vi "8_ВПАнализСтрок.vi"() -> ()   [LabVIEW 2016]
panel:
  out "No Match":bool
  out "Matched Pattern":string
  in  "Password":string
  out "String Subset":string
  in  "Input String":string
  out "Number":dbl
  in  "Number Offset":i16
  in  "Subset Length":i16
  in  "Subset Offset":i16
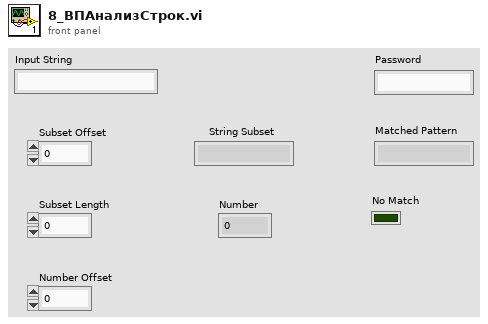
[diagram p1: front panel]
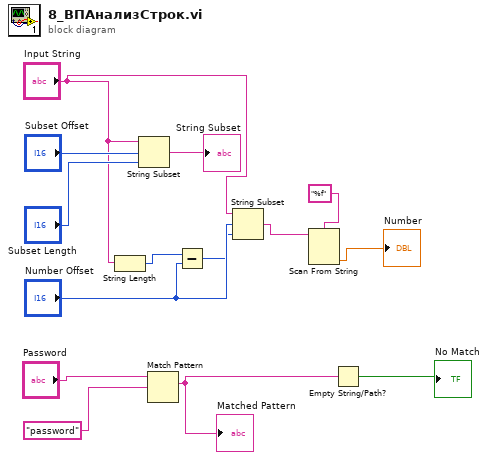
[diagram p0: block diagram]
diagram:
  n1 = String Length(string="Input String") -> (length=w3:i32)
  n2 = String Subset(string="Input String", offset (0)="Subset Offset", length (rest)="Subset Length") -> (substring=→"String Subset":string)
  n3 = Match Pattern(string="Password", regular expression="password") -> (match substring=w5:string)  [unwired: 1 in, 3 out]
  "Matched Pattern" <- w5
  n4 = Subtract(x=w3, y="Number Offset") -> (x-y=w1:i32)
  n5 = String Subset(string="Input String", offset (0)="Number Offset", length (rest)=w1) -> (substring=w10:string)
  n6 = Scan From String(format string="%f", input string=w10) -> (output 1=→"Number":dbl)  [unwired: 3 in, 3 out]
  n7 = Empty String/Path?(string/path=w5) -> (empty?=→"No Match":bool)
